vi "ismatec.vi"() -> ()   [LabVIEW 2015]
uses:
  BERTTA.dll
panel:
  in  "Slide":dbl(slide) scale=0.0..200.0
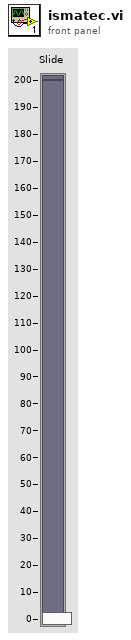
[diagram p1: front panel]
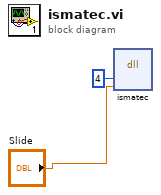
[diagram p0: block diagram]
diagram:
  n1 = dll-call lib="C:/Users/xlaraser/Documents/Visual Studio 2017/Projects/Bertta/BERTTA/Debug/BERTTA.dll" fn="ismatec"("port"=4, "speed"="Slide") -> ()  [unwired: 6 in, 2 out]
